vi "AvRvC_Calc.vi"(11 "data":cluster{"t0":dbl, "df":dbl, "Y":cdb[]}[](array[cluster])) -> (1 "AvC":cluster{"t0":dbl, "df":dbl, "Y":dbl[]}, 3 "AvR":cluster{"t0":dbl, "df":dbl, "Y":dbl[]})   [LabVIEW 2022 SP3]
uses:
  <vilib>/Analysis/5stat.llb/RMS (CDB).vi
  <vilib>/Analysis/baseanly.llb/Mean (CDB).vi
  <vilib>/Analysis/NI_AALPro.lvlib
  <vilib>/Analysis/NI_AALBase.lvlib
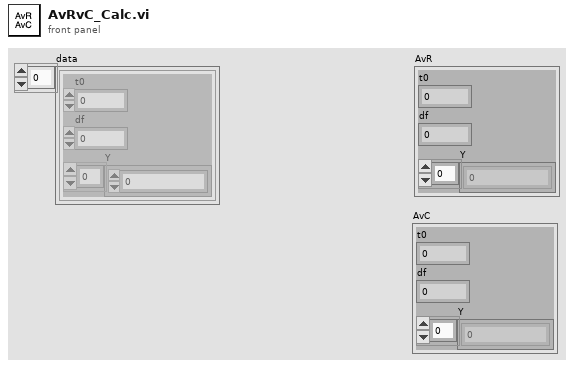
[diagram p1: front panel]
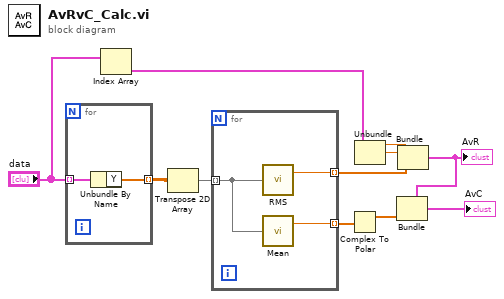
[diagram p0: block diagram]
diagram:
  n1 = for {
    tunnel: "data" -> [w13] mode=indexing
    tunnel: [w12] -> w11 mode=indexing
    n2 = Unbundle By Name(w13) -> ("Y"=w12:cdb[])
  }
  n3 = Index Array(array="data") -> (element=w4:cluster{"t0":dbl, "df":dbl, "Y":cdb[]})  [unwired: 1 in]
  n4 = Transpose 2D Array(2D array=w11) -> (transposed array=w10:cdb[][])
  n5 = for {
    tunnel: w10 -> [w15] mode=indexing
    tunnel: [w16] -> w8 mode=indexing
    tunnel: [w14] -> w7 mode=indexing
    n6 = call-poly <vilib>:"RMS.vi"("X"=w15) -> ("rms value"=w16:dbl)  [unwired: 1 out]
    n7 = call-poly <vilib>:"Mean.vi"("X"=w15) -> ("mean"=w14:cdb)  [unwired: 1 out]
  }
  n8 = Complex To Polar(r * e^(i*theta)=w7) -> (r=w6:dbl[])  [unwired: 1 out]
  n9 = Unbundle(w4) -> ("t0"=w3:dbl, "df"=w2:dbl)  [unwired: 1 out]
  n10 = Bundle("t0"=w3, "df"=w2, w8) -> (w1:cluster{"t0":dbl, "df":dbl, dbl[]})  [unwired: 1 in]
  "AvR" <- w1
  n11 = Bundle(cluster=w1, w6) -> (→"AvC":cluster{"t0":dbl, "df":dbl, dbl[]})  [unwired: 2 in]
